vi "StateClimber.vi"(0 "Master State Out":T1(ring)) -> ()   [LabVIEW 2023]
doc: "This VI performs all of the calculations and decisions related to the swerve drive."
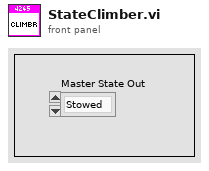
[diagram p1: front panel]
types:
  T1 = enum16{"Stowed", "Balancing", "Scoring", "Hoppering", "Ground", "Shelf"}
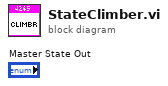
[diagram p0: block diagram]
diagram:
